vi "2.Rtde.vi"() -> ()   [LabVIEW 2022 SP3]
uses:
  UnderAutomation.UniversalRobots/UnderAutomation.UniversalRobots.lvlib
panel:
  in  "SpeedSliderFraction":dbl
  in  "InputIntRegisters.X11":i32
  in  "InputIntRegisters.X10":i32
  in  "SpeedSliderMask":u32
  in  "stop":bool
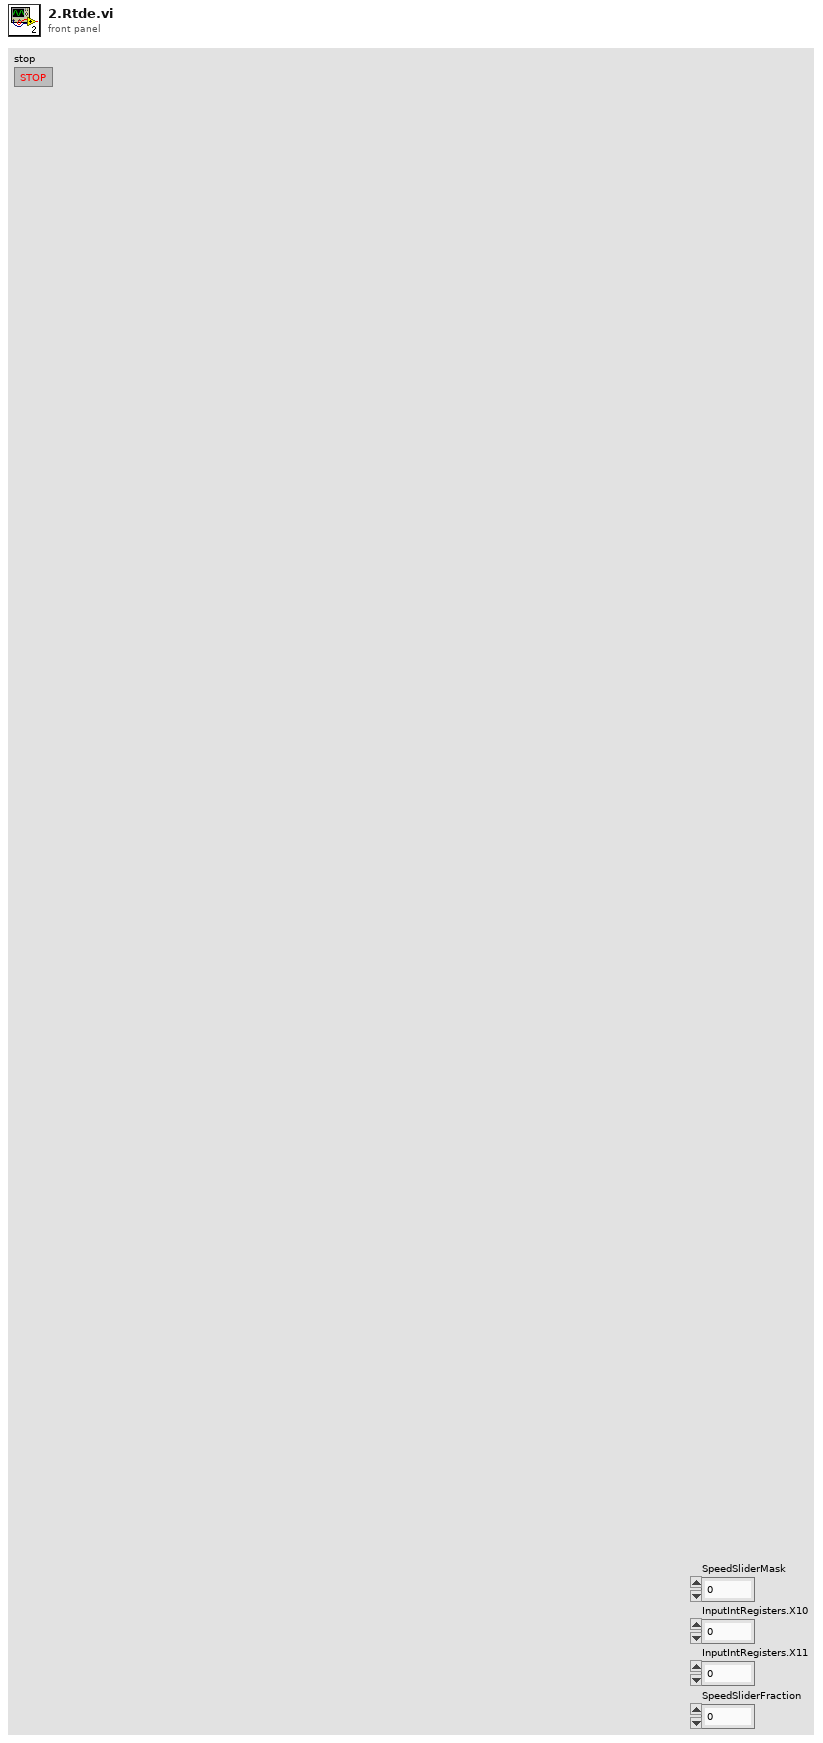
[diagram p1: front panel]
types:
  T1 = cluster{"ConfigurableDigitalOutput":u8, "ConfigurableDigitalOutputMask":u8, "ExternalForceTorque":cluster{"X":dbl, "Y":dbl, "Z":dbl, "Rx":dbl, "Ry":dbl, "Rz":dbl}, "InputBitRegisters":cluster{"X64":bool, "X65":bool, "X66":bool, "X67":bool, "X68":bool, "X69":bool, "X70":bool, "X71":bool, "X72":bool, "X73":bool, "X74":bool, "X75":bool, "X76":bool, "X77":bool, "X78":bool, "X79":bool, "X80":bool, "X81":bool, "X82":bool, "X83":bool, "X84":bool, "X85":bool, "X86":bool, "X87":bool, "X88":bool, "X89":bool, "X90":bool, "X91":bool, "X92":bool, "X93":bool, "X94":bool, "X95":bool, "X96":bool, "X97":bool, "X98":bool, "X99":bool, "X100":bool, "X101":bool, "X102":bool, "X103":bool, "X104":bool, "X105":bool, "X106":bool, "X107":bool, "X108":bool, "X109":bool, "X110":bool, "X111":bool, "X112":bool, "X113":bool, "X114":bool, "X115":bool, "X116":bool, "X117":bool, "X118":bool, "X119":bool, "X120":bool, "X121":bool, "X122":bool, "X123":bool, "X124":bool, "X125":bool, "X126":bool, "X127":bool}, "InputBtRegisters0To31":u32, "InputBtRegisters32To63":u32, "InputDoubleRegisters":cluster{"X0":dbl, "X1":dbl, "X2":dbl, "X3":dbl, "X4":dbl, "X5":dbl, "X6":dbl, "X7":dbl, "X8":dbl, "X9":dbl, "X10":dbl, "X11":dbl, "X12":dbl, "X13":dbl, "X14":dbl, "X15":dbl, "X16":dbl, "X17":dbl, "X18":dbl, "X19":dbl, "X20":dbl, "X21":dbl, "X22":dbl, "X23":dbl, "X24":dbl, "X25":dbl, "X26":dbl, "X27":dbl, "X28":dbl, "X29":dbl, "X30":dbl, "X31":dbl, "X32":dbl, "X33":dbl, "X34":dbl, "X35":dbl, "X36":dbl, "X37":dbl, "X38":dbl, "X39":dbl, "X40":dbl, "X41":dbl, "X42":dbl, "X43":dbl, "X44":dbl, "X45":dbl, "X46":dbl, "X47":dbl}, "InputIntRegisters":cluster{"X0":i32, "X1":i32, "X2":i32, "X3":i32, "X4":i32, "X5":i32, "X6":i32, "X7":i32, "X8":i32, "X9":i32, "X10":i32, "X11":i32, "X12":i32, "X13":i32, "X14":i32, "X15":i32, "X16":i32, "X17":i32, "X18":i32, "X19":i32, "X20":i32, "X21":i32, "X22":i32, "X23":i32, "X24":i32, "X25":i32, "X26":i32, "X27":i32, "X28":i32, "X29":i32, "X30":i32, "X31":i32, "X32":i32, "X33":i32, "X34":i32, "X35":i32, "X36":i32, "X37":i32, "X38":i32, "X39":i32, "X40":i32, "X41":i32, "X42":i32, "X43":i32, "X44":i32, "X45":i32, "X46":i32, "X47":i32}, "SpeedSliderFraction":dbl, "SpeedSliderMask":u32, "StandardAnalogOutput0":dbl, "StandardAnalogOutput1":dbl, "StandardAnalogOutputMask":u8, "StandardAnalogOutputType":u8, "StandardDigitalOutput":u8, "StandardDigitalOutputMask":u8}
  T2 = cluster{"ActualCurrent":cluster{"Base":dbl, "Elbow":dbl, "Shoulder":dbl, "Wrist1":dbl, "Wrist2":dbl, "Wrist3":dbl}, "ActualDigitalInputBits":u64, "ActualDigitalOutputBits":u64, "ActualExecutionTime":dbl, "ActualJointVoltage":cluster{"Base":dbl, "Elbow":dbl, "Shoulder":dbl, "Wrist1":dbl, "Wrist2":dbl, "Wrist3":dbl}, "ActualMainVoltage":dbl, "ActualMomentum":dbl, "ActualQ":cluster{"Base":dbl, "Elbow":dbl, "Shoulder":dbl, "Wrist1":dbl, "Wrist2":dbl, "Wrist3":dbl}, "ActualQd":cluster{"Base":dbl, "Elbow":dbl, "Shoulder":dbl, "Wrist1":dbl, "Wrist2":dbl, "Wrist3":dbl}, "ActualRobotCurrent":dbl, "ActualRobotVoltage":dbl, "ActualTcpForce":cluster{"X":dbl, "Y":dbl, "Z":dbl, "Rx":dbl, "Ry":dbl, "Rz":dbl}, "ActualTcpPose":cluster{"X":dbl, "Y":dbl, "Z":dbl, "Rx":dbl, "Ry":dbl, "Rz":dbl}, "ActualTcpSpeed":cluster{"X":dbl, "Y":dbl, "Z":dbl, "Rx":dbl, "Ry":dbl, "Rz":dbl}, "ActualToolAccelerometer":cluster{"X":dbl, "Y":dbl, "Z":dbl}, "AnalogIOTypes":u32, "ElbowPosition":cluster{"X":dbl, "Y":dbl, "Z":dbl}, "ElbowVelocity":cluster{"X":dbl, "Y":dbl, "Z":dbl}, "Euromap67_24VCurrent":dbl, "Euromap67_24VVoltage":dbl, "Euromap67InputBits":u32, "Euromap67OutputBits":u32, "FTRawWrench":cluster{"X":dbl, "Y":dbl, "Z":dbl, "Rx":dbl, "Ry":dbl, "Rz":dbl}, "InputBitRegisters":cluster{"X64":bool, "X65":bool, "X66":bool, "X67":bool, "X68":bool, "X69":bool, "X70":bool, "X71":bool, "X72":bool, "X73":bool, "X74":bool, "X75":bool, "X76":bool, "X77":bool, "X78":bool, "X79":bool, "X80":bool, "X81":bool, "X82":bool, "X83":bool, "X84":bool, "X85":bool, "X86":bool, "X87":bool, "X88":bool, "X89":bool, "X90":bool, "X91":bool, "X92":bool, "X93":bool, "X94":bool, "X95":bool, "X96":bool, "X97":bool, "X98":bool, "X99":bool, "X100":bool, "X101":bool, "X102":bool, "X103":bool, "X104":bool, "X105":bool, "X106":bool, "X107":bool, "X108":bool, "X109":bool, "X110":bool, "X111":bool, "X112":bool, "X113":bool, "X114":bool, "X115":bool, "X116":bool, "X117":bool, "X118":bool, "X119":bool, "X120":bool, "X121":bool, "X122":bool, "X123":bool, "X124":bool, "X125":bool, "X126":bool, "X127":bool}, "InputBitRegisters0To31":u32, "InputBitRegisters32To63":u32, "InputDoubleRegisters":cluster{"X0":dbl, "X1":dbl, "X2":dbl, "X3":dbl, "X4":dbl, "X5":dbl, "X6":dbl, "X7":dbl, "X8":dbl, "X9":dbl, "X10":dbl, "X11":dbl, "X12":dbl, "X13":dbl, "X14":dbl, "X15":dbl, "X16":dbl, "X17":dbl, "X18":dbl, "X19":dbl, "X20":dbl, "X21":dbl, "X22":dbl, "X23":dbl, "X24":dbl, "X25":dbl, "X26":dbl, "X27":dbl, "X28":dbl, "X29":dbl, "X30":dbl, "X31":dbl, "X32":dbl, "X33":dbl, "X34":dbl, "X35":dbl, "X36":dbl, "X37":dbl, "X38":dbl, "X39":dbl, "X40":dbl, "X41":dbl, "X42":dbl, "X43":dbl, "X44":dbl, "X45":dbl, "X46":dbl, "X47":dbl}, "InputIntRegisters":cluster{"X0":i32, "X1":i32, "X2":i32, "X3":i32, "X4":i32, "X5":i32, "X6":i32, "X7":i32, "X8":i32, "X9":i32, "X10":i32, "X11":i32, "X12":i32, "X13":i32, "X14":i32, "X15":i32, "X16":i32, "X17":i32, "X18":i32, "X19":i32, "X20":i32, "X21":i32, "X22":i32, "X23":i32, "X24":i32, "X25":i32, "X26":i32, "X27":i32, "X28":i32, "X29":i32, "X30":i32, "X31":i32, "X32":i32, "X33":i32, "X34":i32, "X35":i32, "X36":i32, "X37":i32, "X38":i32, "X39":i32, "X40":i32, "X41":i32, "X42":i32, "X43":i32, "X44":i32, "X45":i32, "X46":i32, "X47":i32}, "IOCurrent":dbl, "JointControlOutput":cluster{"Base":dbl, "Elbow":dbl, "Shoulder":dbl, "Wrist1":dbl, "Wrist2":dbl, "Wrist3":dbl}, "JointMode":cluster{"Base":i32, "Elbow":i32, "Shoulder":i32, "Wrist1":i32, "Wrist2":i32, "Wrist3":i32}, "JointTemperatures":cluster{"Base":dbl, "Elbow":dbl, "Shoulder":dbl, "Wrist1":dbl, "Wrist2":dbl, "Wrist3":dbl}, "OutputBitRegisters":cluster{"X64":bool, "X65":bool, "X66":bool, "X67":bool, "X68":bool, "X69":bool, "X70":bool, "X71":bool, "X72":bool, "X73":bool, "X74":bool, "X75":bool, "X76":bool, "X77":bool, "X78":bool, "X79":bool, "X80":bool, "X81":bool, "X82":bool, "X83":bool, "X84":bool, "X85":bool, "X86":bool, "X87":bool, "X88":bool, "X89":bool, "X90":bool, "X91":bool, "X92":bool, "X93":bool, "X94":bool, "X95":bool, "X96":bool, "X97":bool, "X98":bool, "X99":bool, "X100":bool, "X101":bool, "X102":bool, "X103":bool, "X104":bool, "X105":bool, "X106":bool, "X107":bool, "X108":bool, "X109":bool, "X110":bool, "X111":bool, "X112":bool, "X113":bool, "X114":bool, "X115":bool, "X116":bool, "X117":bool, "X118":bool, "X119":bool, "X120":bool, "X121":bool, "X122":bool, "X123":bool, "X124":bool, "X125":bool, "X126":bool, "X127":bool}, "OutputBitRegisters0To31":u32, "OutputBitRegisters32To63":u32, "OutputDoubleRegisters":cluster{"X0":dbl, "X1":dbl, "X2":dbl, "X3":dbl, "X4":dbl, "X5":dbl, "X6":dbl, "X7":dbl, "X8":dbl, "X9":dbl, "X10":dbl, "X11":dbl, "X12":dbl, "X13":dbl, "X14":dbl, "X15":dbl, "X16":dbl, "X17":dbl, "X18":dbl, "X19":dbl, "X20":dbl, "X21":dbl, "X22":dbl, "X23":dbl, "X24":dbl, "X25":dbl, "X26":dbl, "X27":dbl, "X28":dbl, "X29":dbl, "X30":dbl, "X31":dbl, "X32":dbl, "X33":dbl, "X34":dbl, "X35":dbl, "X36":dbl, "X37":dbl, "X38":dbl, "X39":dbl, "X40":dbl, "X41":dbl, "X42":dbl, "X43":dbl, "X44":dbl, "X45":dbl, "X46":dbl, "X47":dbl}, "OutputIntRegisters":cluster{"X0":i32, "X1":i32, "X2":i32, "X3":i32, "X4":i32, "X5":i32, "X6":i32, "X7":i32, "X8":i32, "X9":i32, "X10":i32, "X11":i32, "X12":i32, "X13":i32, "X14":i32, "X15":i32, "X16":i32, "X17":i32, "X18":i32, "X19":i32, "X20":i32, "X21":i32, "X22":i32, "X23":i32, "X24":i32, "X25":i32, "X26":i32, "X27":i32, "X28":i32, "X29":i32, "X30":i32, "X31":i32, "X32":i32, "X33":i32, "X34":i32, "X35":i32, "X36":i32, "X37":i32, "X38":i32, "X39":i32, "X40":i32, "X41":i32, "X42":i32, "X43":i32, "X44":i32, "X45":i32, "X46":i32, "X47":i32}, "Payload":dbl, "PayloadCOG":cluster{"X":dbl, "Y":dbl, "Z":dbl}, "PayloadInertia":cluster{"X":dbl, "Y":dbl, "Z":dbl, "Rx":dbl, "Ry":dbl, "Rz":dbl}, "RobotMode":i32, "RobotStatusBits":u32, "RuntimeState":u32, "SafetyMode":i32, "SafetyStatus":i32, "SafetyStatusBits":u32, "ScriptControlLine":u32, "SpeedScaling":dbl, "StandardAnalogInput0":dbl, "StandardAnalogInput1":dbl, "StandardAnalogOutput0":dbl, "StandardAnalogOutput1":dbl, "TargetCurrent":cluster{"Base":dbl, "Elbow":dbl, "Shoulder":dbl, "Wrist1":dbl, "Wrist2":dbl, "Wrist3":dbl}, "TargetMoment":cluster{"Base":dbl, "Elbow":dbl, "Shoulder":dbl, "Wrist1":dbl, "Wrist2":dbl, "Wrist3":dbl}, "TargetQ":cluster{"Base":dbl, "Elbow":dbl, "Shoulder":dbl, "Wrist1":dbl, "Wrist2":dbl, "Wrist3":dbl}, "TargetQd":cluster{"Base":dbl, "Elbow":dbl, "Shoulder":dbl, "Wrist1":dbl, "Wrist2":dbl, "Wrist3":dbl}, "TargetQdd":cluster{"Base":dbl, "Elbow":dbl, "Shoulder":dbl, "Wrist1":dbl, "Wrist2":dbl, "Wrist3":dbl}, "TargetSpeedFraction":dbl, "TargetTcpPose":cluster{"X":dbl, "Y":dbl, "Z":dbl, "Rx":dbl, "Ry":dbl, "Rz":dbl}, "TargetTcpSpeed":cluster{"X":dbl, "Y":dbl, "Z":dbl, "Rx":dbl, "Ry":dbl, "Rz":dbl}, "TcpForceScalar":dbl, "Timestamp":dbl, "ToolAnalogInput0":dbl, "ToolAnalogInput1":dbl, "ToolAnalogInputTypes":u32, "ToolDigitalOutput0mode":u8, "ToolDigitalOutput1Mode":u8, "ToolMode":u32, "ToolOutputCurrent":dbl, "ToolOutputMode":u8, "ToolOutputVoltage":i32, "ToolTemperature":dbl}
  T3 = cluster{"X":dbl, "Y":dbl, "Z":dbl, "Rx":dbl, "Ry":dbl, "Rz":dbl}
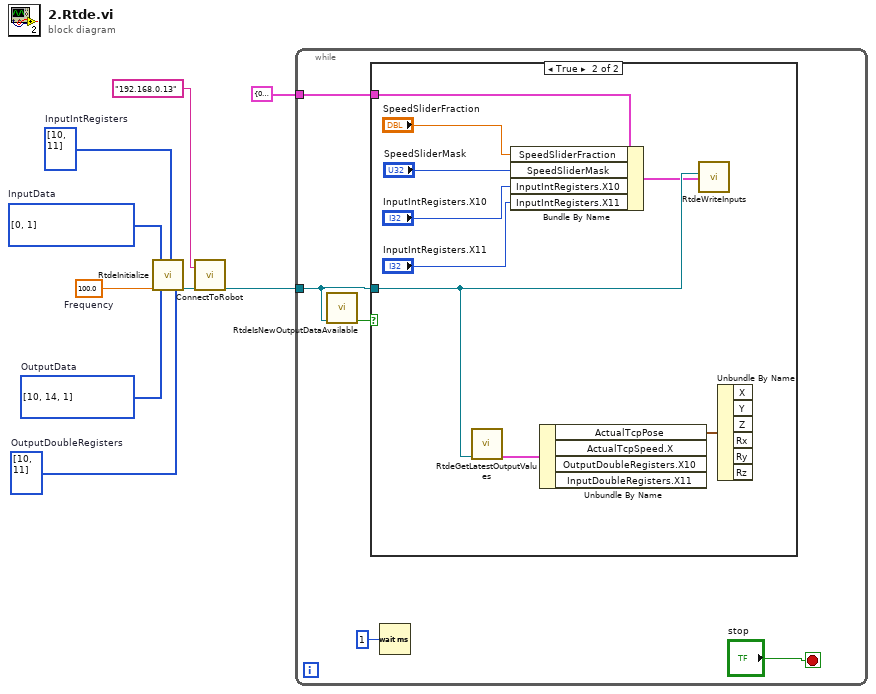
[diagram p0: block diagram]
diagram:
  w2 = i32[] [10, 11]  # OutputDoubleRegisters
  w3 = i32[] [10, 11]  # InputIntRegisters
  w4 = i32[] [0, 1] items=["SpeedSliderMask", "SpeedSliderFraction", "StandardDigitalOutputMask", "ConfigurableDigitalOutputMask", "StandardDigitalOutput", "ConfigurableDigitalOutput", "StandardAnalogOutputMask", "StandardAnalogOutputType", "StandardAnalogOutput0", "StandardAnalogOutput1", "InputBtRegisters0To31", "InputBtRegisters32To63", "InputBitRegisters", "InputIntRegisters", "InputDoubleRegisters", "ExternalForceTorque"]  # InputData
  w5 = 100.0  # Frequency
  w6 = i32[] [10, 14, 1] items=["Timestamp", "TargetQ", "TargetQd", "TargetQdd", "TargetCurrent", "TargetMoment", "ActualQ", "ActualQd", "ActualCurrent", "JointControlOutput", "ActualTcpPose", "ActualTcpSpeed", "ActualTcpForce", "TargetTcpPose", "TargetTcpSpeed", "ActualDigitalInputBits", "JointTemperatures", "ActualExecutionTime", "RobotMode", "JointMode", "SafetyMode", "SafetyStatus", "ActualToolAccelerometer", "SpeedScaling", "TargetSpeedFraction", "ActualMomentum", "ActualMainVoltage", "ActualRobotVoltage", "ActualRobotCurrent", "ActualJointVoltage", "ActualDigitalOutputBits", "RuntimeState", "ElbowPosition", "ElbowVelocity", "RobotStatusBits", "SafetyStatusBits", "AnalogIOTypes", "StandardAnalogInput0", "StandardAnalogInput1", "StandardAnalogOutput0", "StandardAnalogOutput1", "IOCurrent", "Euromap67InputBits", "Euromap67OutputBits", "Euromap67_24VVoltage", "Euromap67_24VCurrent", "ToolMode", "ToolAnalogInputTypes", "ToolAnalogInput0", "ToolAnalogInput1", "ToolOutputVoltage", "ToolOutputCurrent", "ToolTemperature", "TcpForceScalar", "OutputBitRegisters0To31", "OutputBitRegisters32To63", "OutputBitRegisters", "OutputIntRegisters", "OutputDoubleRegisters", "InputBitRegisters0To31", "InputBitRegisters32To63", "InputBitRegisters", "InputIntRegisters", "InputDoubleRegisters", "ToolOutputMode", "ToolDigitalOutput0mode", "ToolDigitalOutput1Mode", "Payload", "PayloadCOG", "PayloadInertia", "ScriptControlLine", "FTRawWrench"]  # OutputData
  n1 = call "RtdeInitialize.vi"("Frequency"=w5, "InputData"=w4, "OutputData"=w6, "InputIntRegisters"=w3, "OutputDoubleRegisters"=w2) -> ("RTDE Connect Parameters"=w7:refnum<k24>)  [unwired: 13 in, 1 out]
  n2 = call "ConnectToRobot.vi"("ip"="192.168.0.13", "RTDE Connect Parameters"=w7) -> ("Rtde"=w8:refnum<k24>)  [unwired: 12 in, 5 out]
  n3 = while {
    tunnel: w8 -> [w11]
    tunnel: T1 {"ConfigurableDigitalOutput"=0, "ConfigurableDigitalOutputMask"=0, "ExternalForceTorque"={"X"=0.0, "Y"=0.0, "Z"=0.0, "Rx"=0.0, "Ry"=0.0, "Rz"=0.0}, "InputBitRegisters"={"X64"=FALSE, "X65"=FALSE, "X66"=FALSE, "X67"=FALSE, "X68"=FALSE, "X69"=FALSE, "X70"=FALSE, "X71"=FALSE, "X72"=FALSE, "X73"=FALSE, "X74"=FALSE, "X75"=FALSE, "X76"=FALSE, "X77"=FALSE, "X78"=FALSE, "X79"=FALSE, "X80"=FALSE, "X81"=FALSE, "X82"=FALSE, "X83"=FALSE, "X84"=FALSE, "X85"=FALSE, "X86"=FALSE, "X87"=FALSE, "X88"=FALSE, "X89"=FALSE, "X90"=FALSE, "X91"=FALSE, "X92"=FALSE, "X93"=FALSE, "X94"=FALSE, "X95"=FALSE, "X96"=FALSE, "X97"=FALSE, "X98"=FALSE, "X99"=FALSE, "X100"=FALSE, "X101"=FALSE, "X102"=FALSE, "X103"=FALSE, "X104"=FALSE, "X105"=FALSE, "X106"=FALSE, "X107"=FALSE, "X108"=FALSE, "X109"=FALSE, "X110"=FALSE, "X111"=FALSE, "X112"=FALSE, "X113"=FALSE, "X114"=FALSE, "X115"=FALSE, "X116"=FALSE, "X117"=FALSE, "X118"=FALSE, "X119"=FALSE, "X120"=FALSE, "X121"=FALSE, "X122"=FALSE, "X123"=FALSE, "X124"=FALSE, "X125"=FALSE, "X126"=FALSE, "X127"=FALSE}, "InputBtRegisters0To31"=0, "InputBtRegisters32To63"=0, "InputDoubleRegisters"={"X0"=0.0, "X1"=0.0, "X2"=0.0, "X3"=0.0, "X4"=0.0, "X5"=0.0, "X6"=0.0, "X7"=0.0, "X8"=0.0, "X9"=0.0, "X10"=0.0, "X11"=0.0, "X12"=0.0, "X13"=0.0, "X14"=0.0, "X15"=0.0, "X16"=0.0, "X17"=0.0, "X18"=0.0, "X19"=0.0, "X20"=0.0, "X21"=0.0, "X22"=0.0, "X23"=0.0, "X24"=0.0, "X25"=0.0, "X26"=0.0, "X27"=0.0, "X28"=0.0, "X29"=0.0, "X30"=0.0, "X31"=0.0, "X32"=0.0, "X33"=0.0, "X34"=0.0, "X35"=0.0, "X36"=0.0, "X37"=0.0, "X38"=0.0, "X39"=0.0, "X40"=0.0, "X41"=0.0, "X42"=0.0, "X43"=0.0, "X44"=0.0, "X45"=0.0, "X46"=0.0, "X47"=0.0}, "InputIntRegisters"={"X0"=0, "X1"=0, "X2"=0, "X3"=0, "X4"=0, "X5"=0, "X6"=0, "X7"=0, "X8"=0, "X9"=0, "X10"=0, "X11"=0, "X12"=0, "X13"=0, "X14"=0, "X15"=0, "X16"=0, "X17"=0, "X18"=0, "X19"=0, "X20"=0, "X21"=0, "X22"=0, "X23"=0, "X24"=0, "X25"=0, "X26"=0, "X27"=0, "X28"=0, "X29"=0, "X30"=0, "X31"=0, "X32"=0, "X33"=0, "X34"=0, "X35"=0, "X36"=0, "X37"=0, "X38"=0, "X39"=0, "X40"=0, "X41"=0, "X42"=0, "X43"=0, "X44"=0, "X45"=0, "X46"=0, "X47"=0}, "SpeedSliderFraction"=0.0, "SpeedSliderMask"=0, "StandardAnalogOutput0"=0.0, "StandardAnalogOutput1"=0.0, "StandardAnalogOutputMask"=0, "StandardAnalogOutputType"=0, "StandardDigitalOutput"=0, "StandardDigitalOutputMask"=0} ("Data") -> [w10]
    stop <- "stop" stop-if-true
    n4 = call "RtdeIsNewOutputDataAvailable.vi"("Rtde"=w11) -> ("Data available"=w12:bool)  [unwired: 9 in, 1 out]
    n5 = case shown="True" w12 {
      tunnel: w11 -> [_ w21]
      tunnel: w10 -> [_ w20]
      frame False {
      }
      frame True {
        n6 = call "RtdeGetLatestOutputValues.vi"("Rtde"=w21) -> ("Data"=w23:T2)  [unwired: 9 in, 1 out]
        n7 = Bundle By Name(cluster=w20, "SpeedSliderFraction"="SpeedSliderFraction", "SpeedSliderMask"="SpeedSliderMask", "InputIntRegisters.X10"="InputIntRegisters.X10", "InputIntRegisters.X11"="InputIntRegisters.X11") -> (w19:T1)
        n8 = Unbundle By Name(w23) -> ("ActualTcpPose"=w22:T3)  [unwired: 3 out]
        n9 = call "RtdeWriteInputs.vi"("Data"=w19, "Rtde"=w21) -> ()  [unwired: 9 in, 1 out]
        n10 = Unbundle By Name(w22) -> ()  [unwired: 6 out]
      }
    }
    n11 = Wait (ms)(milliseconds to wait=u32 1) -> ()  [unwired: 1 out]
  }
